vi "LAUDA_STEPCONTROL07.vi"(10 "step":dbl, 11 "pause":i16) -> (0 "Boolean 13":bool, 1 "Boolean 6":bool, 2 "Boolean 5":bool, 3 "Boolean 4":bool, 4 "Boolean 7":bool, 5 "Boolean 12":bool)   [LabVIEW 2015]
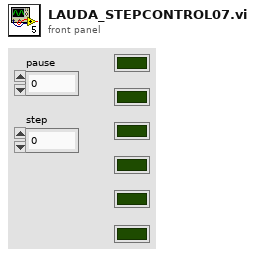
[diagram p1: front panel]
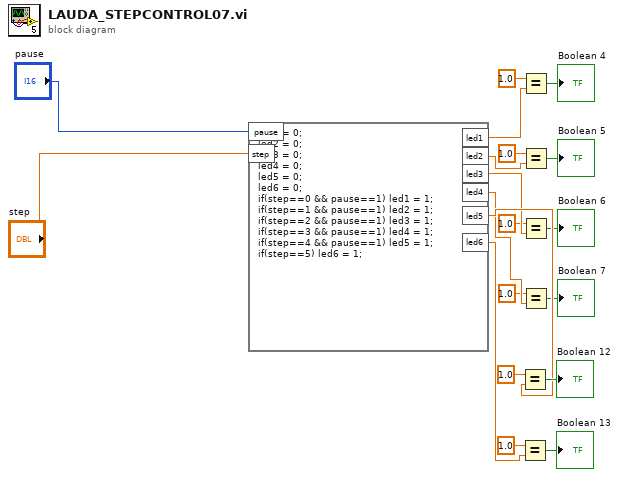
[diagram p0: block diagram]
diagram:
  n1 = formula code="led1 = 0;\nled2 = 0;\nled3 = 0;\nled4 = 0;\nled5 = 0;\nled6 = 0;\nif(step==0 && pause==1) led1 = 1;\nif(step==1 && pause==1) led2 = 1;\nif(step==2 && pause==1) led3 = 1;\nif(step==3 && pause==1) led4 = 1;\nif(step==4 && pause==1) led5 = 1;\nif(step==5) led6 = 1;"("step"="step", "pause"="pause") -> ("led1"=w6:dbl, "led2"=w10:dbl, "led3"=w12:dbl, "led4"=w14:dbl, "led5"=w19:dbl, "led6"=w1:dbl)
  n2 = Equal?(x=1.0, y=w19) -> (x = y?=→"Boolean 12":bool)
  n3 = Equal?(x=1.0, y=w1) -> (x = y?=→"Boolean 13":bool)
  n4 = Equal?(x=1.0, y=w6) -> (x = y?=→"Boolean 4":bool)
  n5 = Equal?(x=1.0, y=w10) -> (x = y?=→"Boolean 5":bool)
  n6 = Equal?(x=1.0, y=w12) -> (x = y?=→"Boolean 6":bool)
  n7 = Equal?(x=1.0, y=w14) -> (x = y?=→"Boolean 7":bool)
